vi "average.vi"(10 "Numeric in":dbl, 11 "Numeric 3":dbl) -> (3 "Numeric out":dbl)   [LabVIEW 2014]
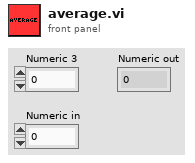
[diagram p1: front panel]
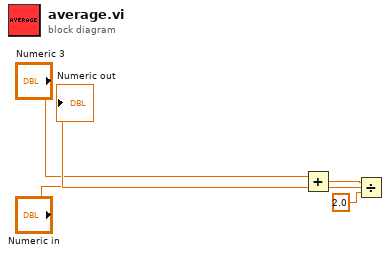
[diagram p0: block diagram]
diagram:
  n1 = Add(x="Numeric 3", y="Numeric in") -> (x+y=w3:dbl)
  n2 = Divide(x=w3, y=2.0) -> (x/y=→"Numeric out":dbl)
